vi "Delete Linked List.vi"(8 "error in (no error)":errorcluster, 10 "Unique ID":string, 11 "Linked List in":refnum<class "Linked List.lvclass">) -> (0 "error out":errorcluster, 3 "Linked List out":refnum<class "Linked List.lvclass">)   [LabVIEW 2019, in "Linked Lists.lvlib" / "Linked List.lvclass"]
uses:
  <vilib>/gpm_packages/@cs/linked-list/Source/Linked List/Linked List/Linked List.lvclass
  <vilib>/gpm_packages/@cs/linked-list/Source/Linked List/Linked List Definition/Linked List Definition.lvclass
  <vilib>/gpm_packages/@cs/linked-list/Source/Linked List/Linked List/Linked List.lvclass/Linked List.ctl
  <vilib>/gpm_packages/@cs/lookup-table/Source/LookupTable/LookupTable.lvclass/LookupTable.ctl
  f81a2cb2-fd58-4fb6-b33e-35a0f783fbf4.vi
  a148ee24-9514-4401-a906-8a1f216a6b60.vi
  168ed26c-b9b9-4500-84eb-805c64e5d81e.vi
  <vilib>/gpm_packages/@cs/lookup-table/Source/LookupTable/Read Table Reference.vi
  f81a2cb2-fd58-4fb6-b33e-35a0f783fbf4.vi/14737446-9f6a-49d0-83e8-d5b952631ac1.vi
  <vilib>/gpm_packages/@cs/lookup-table/Source/LookupTable/LookupTable.lvclass
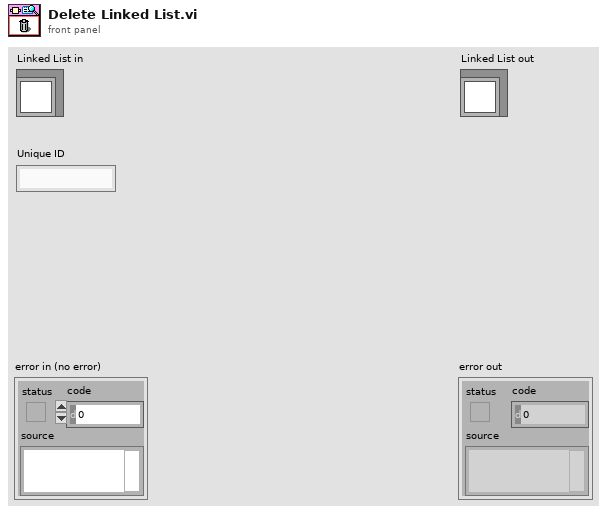
[diagram p1: front panel]
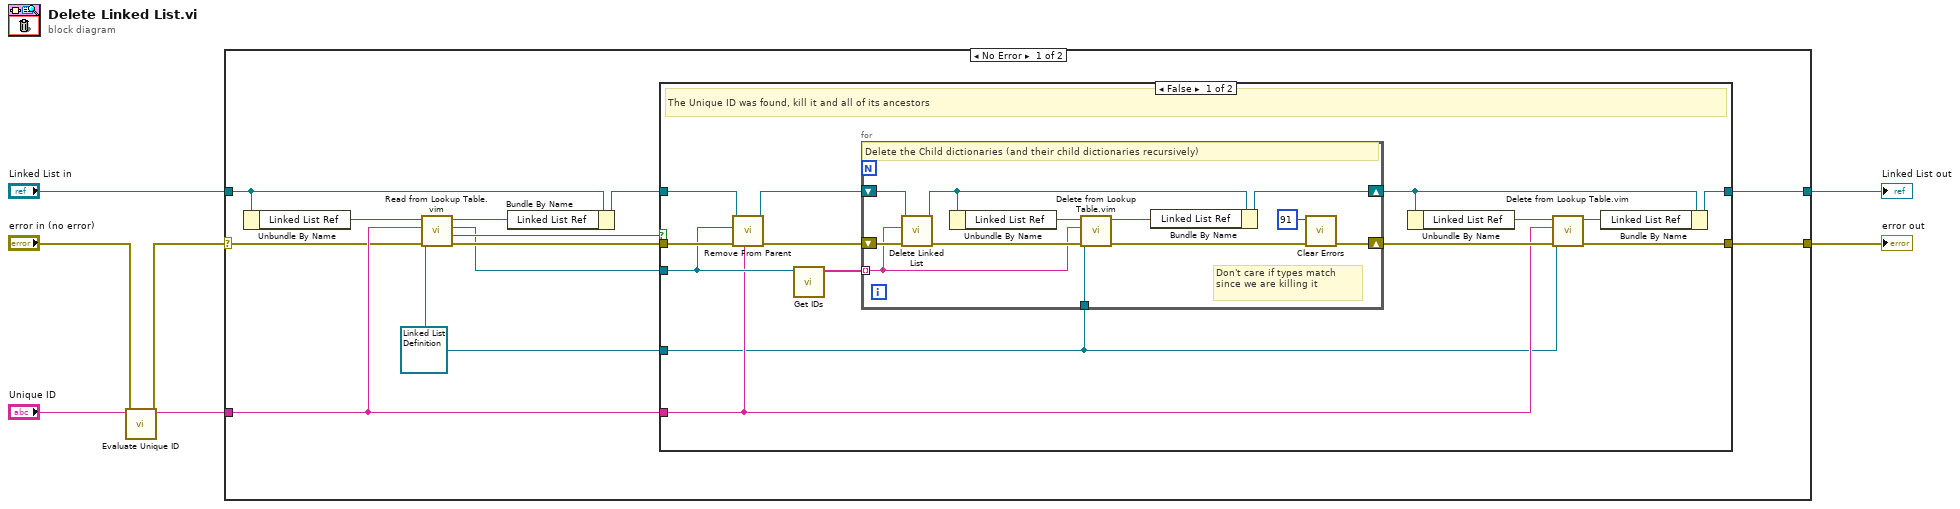
[diagram p0: block diagram]
diagram:
  n1 = call <vilib>:"Evaluate Unique ID.vi"("error in (no error)"="error in (no error)", "Unique ID"="Unique ID") -> ("error out"=w4:errorcluster, "Unique ID Out"=w6:string)  [unwired: 8 in]
  n2 = case shown="No Error" w4 {
    selector: w4 -> [w13 w48]
    tunnel: w6 -> [w14 _]
    tunnel: "Linked List in" -> [w12 w49]
    tunnel: [w9 w49] -> w2
    tunnel: [w8 w48] -> w1
    frame No Error {
      w10 = refnum<class "Linked List Definition.lvclass"> refnum ("Linked List.lvlib:Linked List Definition.lvclass")
      n3 = Unbundle By Name(w12) -> ("Linked List Ref"=w19:refnum<data-value>)
      n4 = call "Read from Lookup Table.vim"("error in (no error)"=w13, "Type"=w10, "Item Name"=w14, "LookupTable Reference"=w19) -> ("error out"=w16:errorcluster, "Not Found?"=w17:bool, "Value"=w15:refnum<class "Linked List Definition.lvclass">, "LookupTable Reference Out"=w18:refnum<data-value>)  [unwired: 4 in]
      n5 = Bundle By Name(cluster=w12, "Linked List Ref"=w18) -> (w11:refnum<class "Linked List.lvclass">)
      n6 = case shown="False" w17 {
        tunnel: w16 -> [w33 w47]
        tunnel: w15 -> [w32 _]
        tunnel: w14 -> [w25 _]
        tunnel: w11 -> [w31 w46]
        tunnel: w10 -> [w24 _]
        tunnel: [w21 w46] -> w9
        tunnel: [w20 w47] -> w8
        frame False {
          # "The Unique ID was found, kill it and all of its ancestors"
          n7 = call <vilib>:"Remove From Parent.vi"("Unique ID"=w25, "error in (no error)"=w33, "Linked List Definition"=w32, "Linked List in"=w31) -> ("error out"=w28:errorcluster, "Linked List out"=w30:refnum<class "Linked List.lvclass">)  [unwired: 6 in]
          n8 = call <vilib>:"Get IDs.vi"("Linked List Definition in"=w32) -> ("Child IDs"=w29:string[])  [unwired: 8 in, 2 out]
          n9 = for {
            shift-right: [w38] -> w22
            shift-left: w30 -> [w35]
            tunnel: w29 -> [w42] mode=indexing
            shift-right: [w37] -> w27
            shift-left: w28 -> [w45]
            tunnel: w24 -> [w41]
            # "Don't care if types match\nsince we are killing it"
            # "Delete the Child dictionaries (and their child dictionaries recursively)"
            n10 = call-dynamic "Delete Linked List.vi"("error in (no error)"=w45, "Unique ID"=w42, "Linked List in"=w35) -> ("error out"=w43:errorcluster, "Linked List out"=w34:refnum<class "Linked List.lvclass">)  [unwired: 7 in]
            n11 = Unbundle By Name(w34) -> ("Linked List Ref"=w44:refnum<data-value>)
            n12 = call "Delete from Lookup Table.vim"("error in (no error)"=w43, "Confirm Type"=w41, "Item Name"=w42, "LookupTable Reference"=w44) -> ("error out"=w40:errorcluster, "LookupTable Reference Out"=w39:refnum<data-value>)  [unwired: 5 in, 1 out]
            n13 = Bundle By Name(cluster=w34, "Linked List Ref"=w39) -> (w38:refnum<class "Linked List.lvclass">)
            n14 = call <vilib>:"Clear Errors.vi"("error in (no error)"=w40, "specific error code to clear (0: all)"=91) -> ("error out"=w37:errorcluster)  [unwired: 4 in, 1 out]
          }
          n15 = Unbundle By Name(w22) -> ("Linked List Ref"=w26:refnum<data-value>)
          n16 = call "Delete from Lookup Table.vim"("error in (no error)"=w27, "Confirm Type"=w24, "Item Name"=w25, "LookupTable Reference"=w26) -> ("error out"=w20:errorcluster, "LookupTable Reference Out"=w23:refnum<data-value>)  [unwired: 5 in, 1 out]
          n17 = Bundle By Name(cluster=w22, "Linked List Ref"=w23) -> (w21:refnum<class "Linked List.lvclass">)
        }
        frame True {
          # "The Unique ID was not found in the dictionary"
        }
      }
    }
    frame Error {
    }
  }
  "error out" <- w1
  "Linked List out" <- w2
